vi "Filter String.vi"(8 "error in (no error)":errorcluster, 9 "Actual Column":i32, 10 "Filter String":string, 11 "Message Log in":refnum<class "Message Log.lvclass">) -> (0 "error out":errorcluster, 3 "Message Log out":refnum<class "Message Log.lvclass">)   [LabVIEW 2017, in "Message Log.lvclass"]
uses:
  Message Log.lvclass
  <vilib>/Utility/miscctls.llb/LVRowAndColumnUnsignedTypeDef.ctl
  Message Log Filter Data.ctl
  Message Log Columns.ctl
  String Filter Type.ctl
  Message Log.lvclass/Message Log.ctl
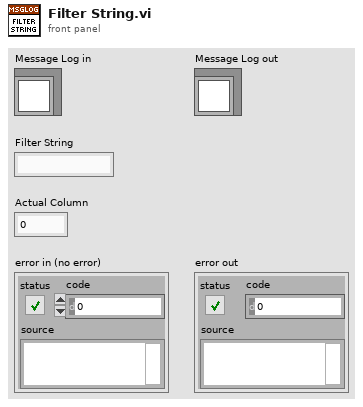
[diagram p1: front panel]
types:
  T1 = typedef "Message Log.lvclass/Message Log Filter Data.ctl" = cluster{"Element":string, "Column":T2, "Filter Type":T3}
  T2 = typedef "Message Log.lvclass/Message Log Columns.ctl" = enum16{"Count (sec)", "Time/Date", "Enque Worker", "Enque Case", "Deque Worker", "Deque Case", "Priority", "Message"}
  T3 = typedef "Message Log.lvclass/String Filter Type.ctl" = enum16{"string only", "match pattern"}
  T4 = typedef "LVRowAndColumnUnsignedTypeDef.ctl" = cluster{"Row":u32, "Column":u32}
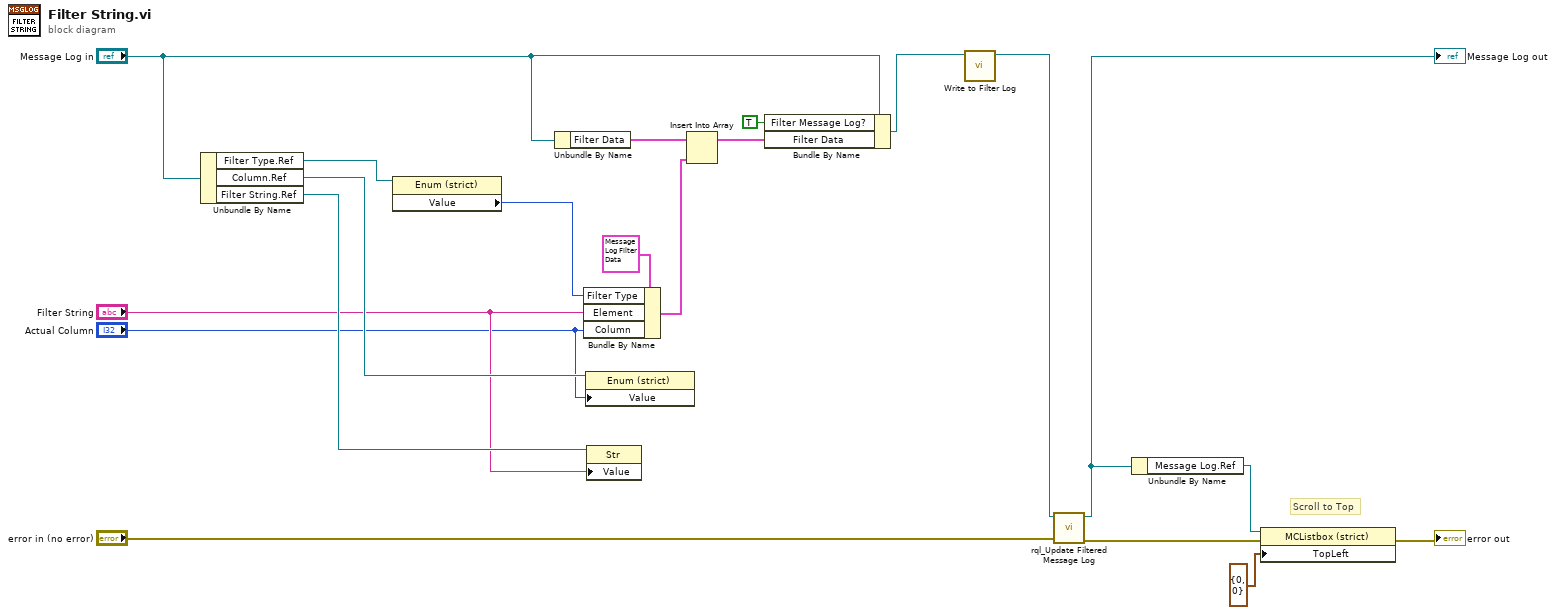
[diagram p0: block diagram]
diagram:
  # "Scroll to Top"
  n1 = Unbundle By Name("Message Log in") -> ("Filter Type.Ref"=w10:refnum<vi>, "Column.Ref"=w9:refnum<vi>, "Filter String.Ref"=w7:refnum<vi>)
  n2 = property class="Enum (strict)"(reference=w10) -> ("Value"=w8:enum16{"string only", "match pattern"})  [unwired: 1 in, 2 out]
  n3 = Unbundle By Name("Message Log in") -> ("Filter Data"=w15:T1[])
  n4 = Bundle By Name(cluster=T1 {"Element"="", "Column"=enum."Count (sec)", "Filter Type"=enum."string only"} ("Message Log Filter Data"), "Filter Type"=w8, "Element"="Filter String", "Column"="Actual Column") -> (w16:T1)
  n5 = property class="Enum (strict)"(reference=w9, "Value"="Actual Column") -> ()  [unwired: 1 in, 2 out]
  n6 = property class="Str"(reference=w7, "Value"="Filter String") -> ()  [unwired: 1 in, 2 out]
  n7 = Insert Into Array(array=w15, new element=w16) -> (w14:T1[])  [unwired: 1 in]
  n8 = Bundle By Name(cluster="Message Log in", "Filter Message Log?"=TRUE, "Filter Data"=w14) -> (w4:refnum<class "Message Log.lvclass">)
  n9 = call "Write to Filter Log.vi"("Message Log in"=w4) -> ("Message Log out"=w19:refnum<class "Message Log.lvclass">)  [unwired: 9 in, 1 out]
  n10 = call "rql_Update Filtered Message Log.vi"("error in"="error in (no error)", "Message Log in"=w19) -> ("error out"=w13:errorcluster, "dup Message Log out"=w3:refnum<class "Message Log.lvclass">)  [unwired: 8 in]
  "Message Log out" <- w3
  n11 = Unbundle By Name(w3) -> ("Message Log.Ref"=w11:refnum<vi>)
  n12 = property class="MCListbox (strict)"(reference=w11, error in=w13, "TopLeft"=T4 {"Row"=0, "Column"=0} ("Top Left Visible Cell")) -> (error out=→"error out":errorcluster)  [unwired: 1 out]
